vi "SlotValidationA1.vi"(10 "EdgeSlotSides":T3[](array[typedef]) {"Distance (Real-World)" format="%.2f"; "Location (Real-World)"."Y" format="%.2g"; "Location (Real-World)"."X" format="%.2f"; "Noise" format="%.2f"; "Location (Pixel)"."Y" format="%.2g"; "Location (Pixel)"."X" format="%.2f"; "Strength" format="%.2f"; "Distance (Pixel)" format="%.2f"}, 11 "ImageIn":T2) -> (2 "槽点":T1(array[cluster]), 3 "ImageOut":T2)   [LabVIEW 2018]
uses:
  <vilib>/vision/Measure.llb/Edge New.ctl
  <vilib>/vision/Image Controls.llb/IMAQ Image.ctl
  <vilib>/vision/NI_Vision_Development_Module.lvlib
panel:
  out "error in (no error) 2":errorcluster caption="error in (no error)"
  in  "验证取点位置":u32 format="%x"
  in  "error in (no error)":errorcluster
  out "Display Image 3":T2(plugin-control)
  in  "限度-槽内平均亮度-上限":sgl=25.0
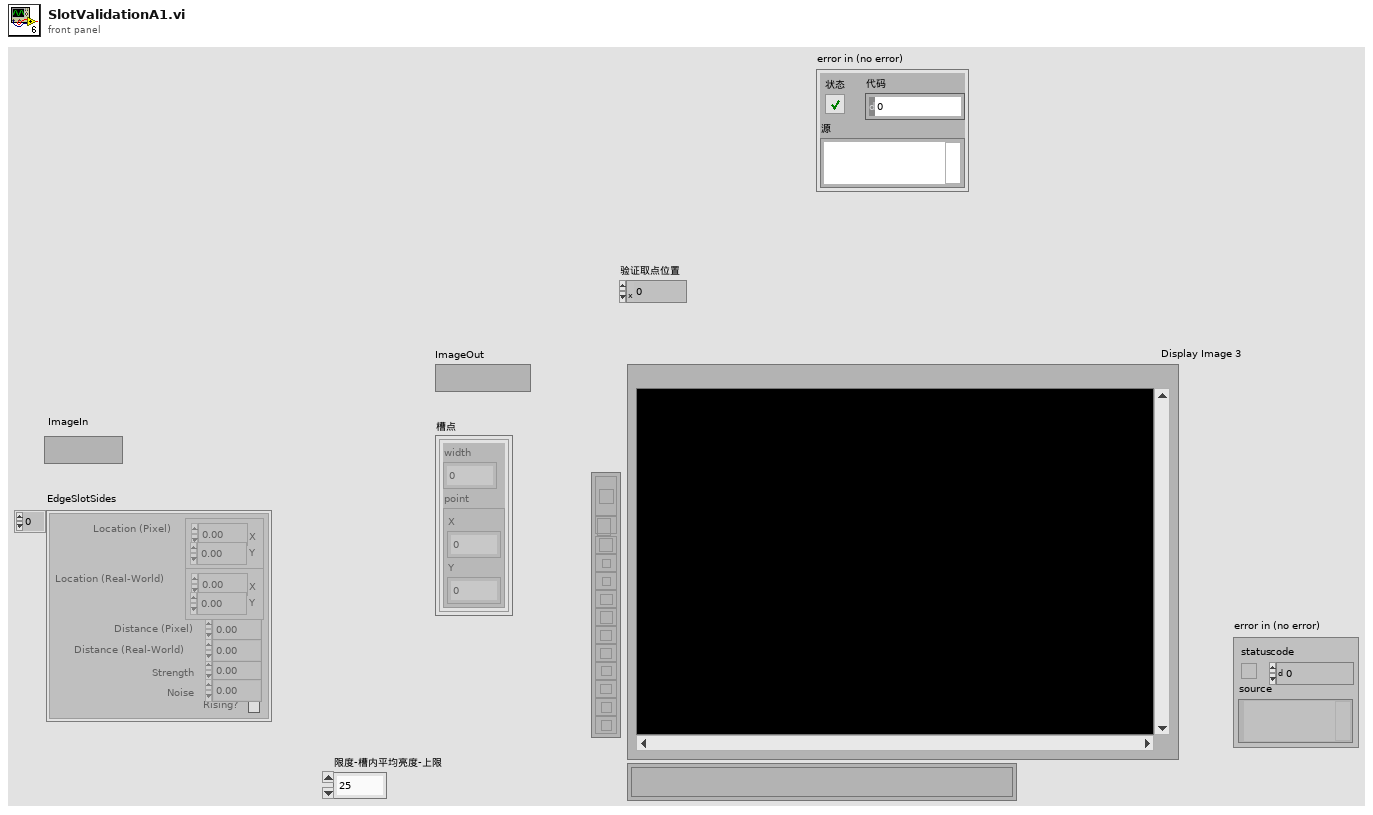
[diagram p1: front panel]
types:
  T1 = cluster{"width":sgl, "point":cluster{"X":sgl, "Y":sgl}}[]
  T2 = typedef "IMAQ Image.ctl" = refnum<image>
  T3 = typedef "Edge New.ctl" = cluster{"Location (Pixel)":cluster{"X":sgl, "Y":sgl}, "Location (Real-World)":cluster{"X":sgl, "Y":sgl}, "Distance (Pixel)":dbl, "Distance (Real-World)":dbl, "Strength":dbl, "Noise":dbl, "Rising?":bool}
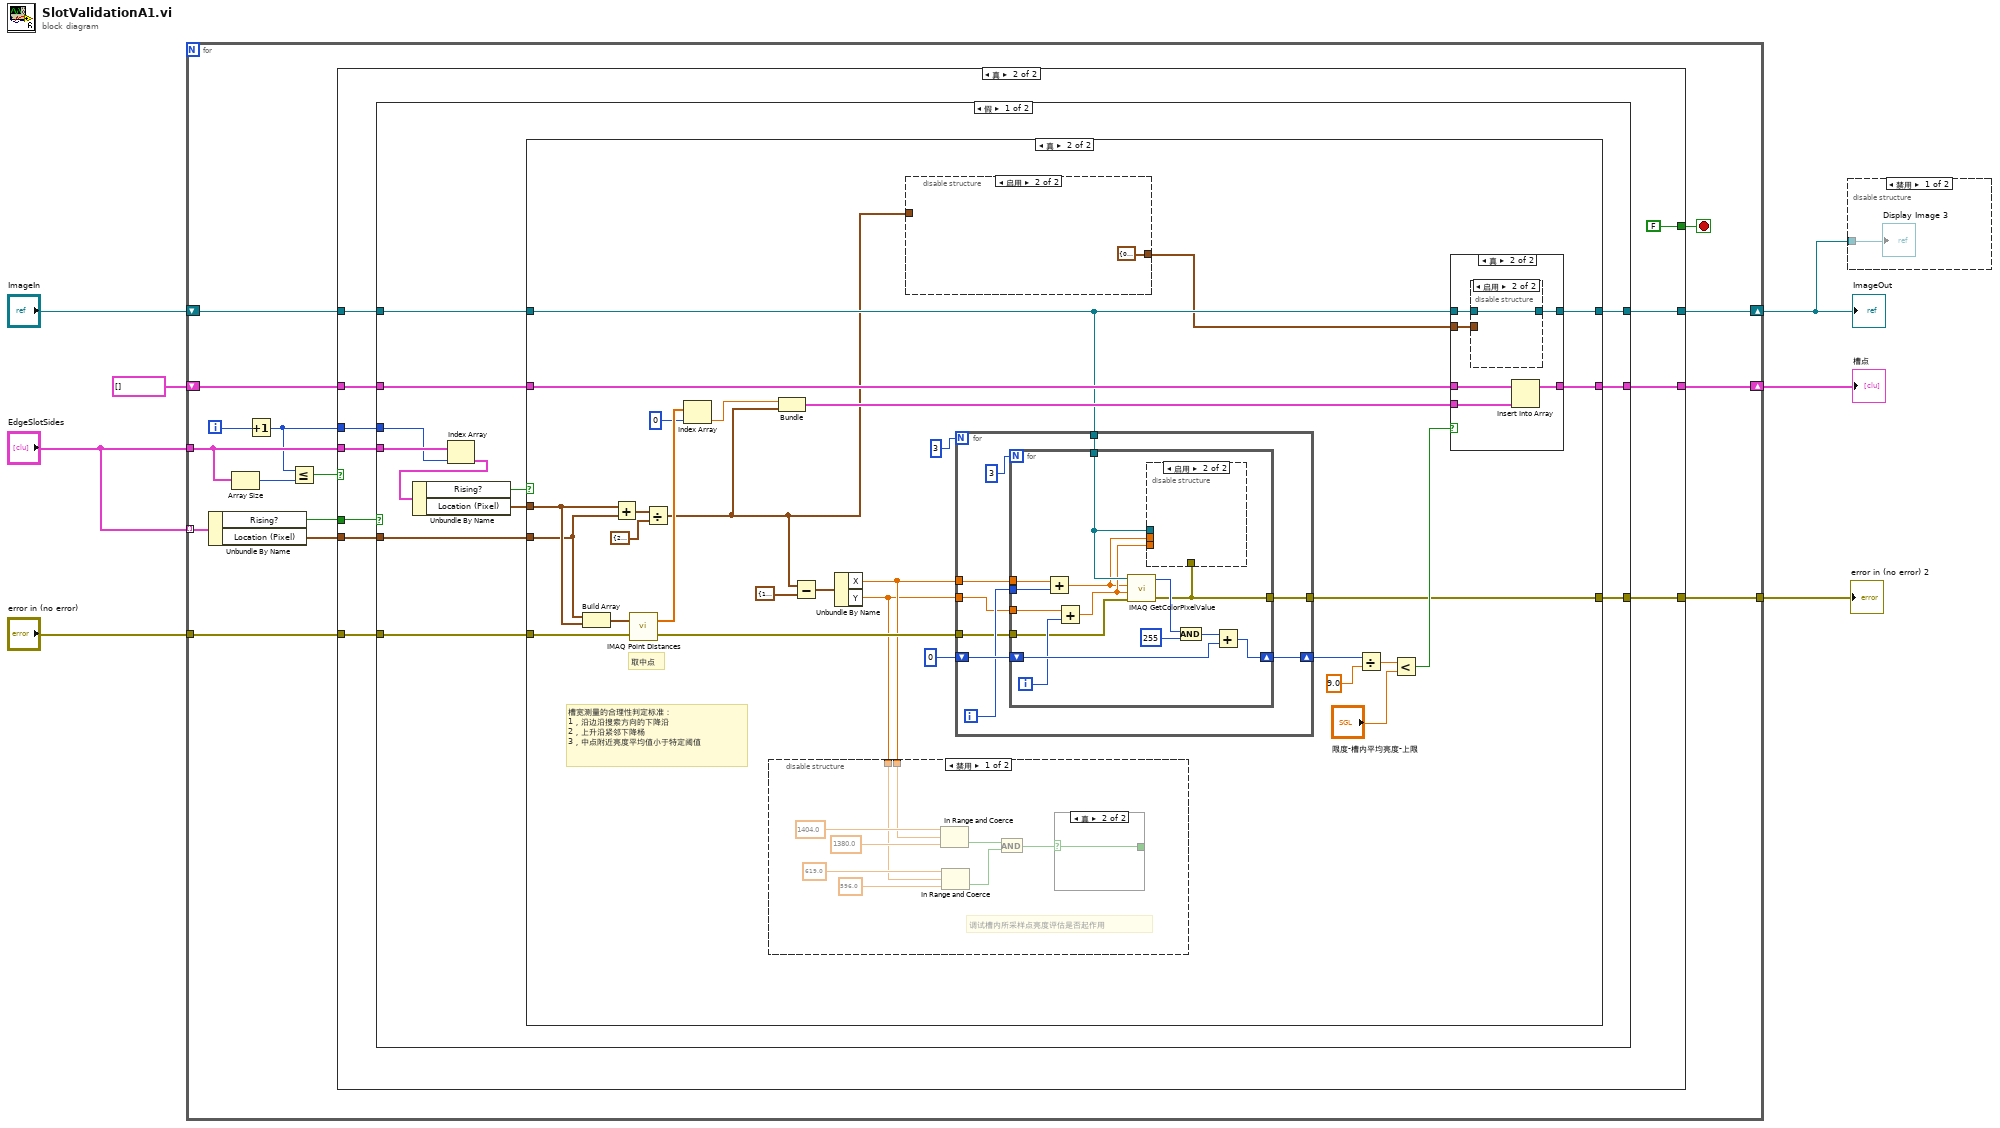
[diagram p0: block diagram]
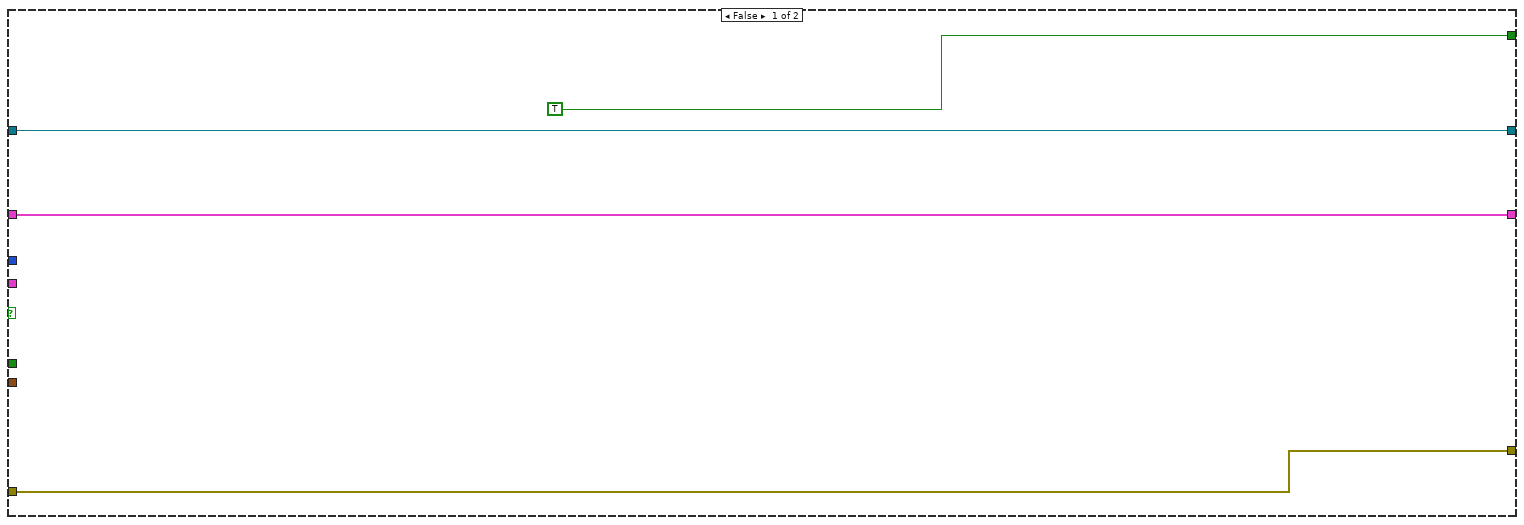
[diagram p3: hidden frame]
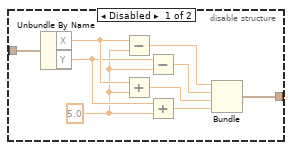
[diagram p7: hidden frame]
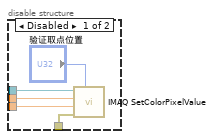
[diagram p8: hidden frame]
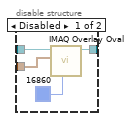
[diagram p10: hidden frame]
diagram:
  n1 = for {
    tunnel: "EdgeSlotSides" -> [w22] mode=indexing
    tunnel: "EdgeSlotSides" -> [w18]
    shift-right: [w13] -> w3
    shift-left: T1 [] ("初始化的数组") -> [w14]
    shift-right: [w11] -> w4
    shift-left: "ImageIn" -> [w12]
    tunnel: "error in (no error)" -> [w9]
    tunnel: [w8] -> w1
    i -> [w19]
    stop <- w15 stop-if-true
    n2 = Unbundle By Name(w22) -> ("Rising?"=w21:bool, "Location (Pixel)"=w20:cluster{"X":sgl, "Y":sgl})
    n3 = Array Size(array=w18) -> (size(s)=w17:i32)
    n4 = Increment(x=w19) -> (x+1=w10:i32)
    n5 = Less Or Equal?(x=w10, y=w17) -> (x <= y?=w16:bool)
    n6 = case shown="真" w16 {
      tunnel: w18 -> [_ w37]
      tunnel: w21 -> [_ w36]
      tunnel: w20 -> [_ w35]
      tunnel: [TRUE FALSE] -> w15
      tunnel: w14 -> [w25 w33]
      tunnel: [w25 w32] -> w13
      tunnel: w12 -> [w24 w31]
      tunnel: [w24 w30] -> w11
      tunnel: w10 -> [_ w29]
      tunnel: w9 -> [w23 w28]
      tunnel: [w23 w27] -> w8
      frame False {
      }
      frame True {
        n7 = case shown="假" w36 {
          tunnel: w37 -> [w49 _]
          tunnel: w35 -> [w45 _]
          tunnel: w33 -> [w44 w146]
          tunnel: [w43 w146] -> w32
          tunnel: w31 -> [w42 w145]
          tunnel: [w41 w145] -> w30
          tunnel: w29 -> [w40 _]
          tunnel: w28 -> [w39 w144]
          tunnel: [w38 w144] -> w27
          frame False {
            n8 = Index Array(array=w49, index=w40) -> (element=w48:T3)
            n9 = Unbundle By Name(w48) -> ("Rising?"=w47:bool, "Location (Pixel)"=w46:cluster{"X":sgl, "Y":sgl})
            n10 = case shown="真" w47 {
              tunnel: w46 -> [_ w69]
              tunnel: w45 -> [_ w68]
              tunnel: w44 -> [w52 w81]
              tunnel: [w52 w80] -> w43
              tunnel: w42 -> [w51 w62]
              tunnel: [w51 w61] -> w41
              tunnel: w39 -> [w50 w60]
              tunnel: [w50 w56] -> w38
              frame False {
              }
              frame True {
                # "槽宽测量的合理性判定标准：\n1，沿边沿搜索方向的下降沿\n2，上升沿紧邻下降杨\n3，中点附近亮度平均值小于特定阈值"
                # "取中点"
                n11 = Build Array(w68, w69) -> (w67:cluster{"X":sgl, "Y":sgl}[])
                n12 = Add(x=w69, y=w68) -> (x+y=w79:cluster{"X":sgl, "Y":sgl})
                n13 = call "IMAQ Point Distances"("Points"=w67, "error in (no error)"=w60) -> ("Distances"=w65:sgl[], "error out"=w59:errorcluster)  [unwired: 3 in]
                n14 = Divide(x=w79, y=cluster{"X":sgl, "Y":sgl} {"X"=2.0, "Y"=2.0} ("Location (Pixel)")) -> (x/y=w55:cluster{"X":sgl, "Y":sgl})
                n15 = Index Array(array=w65, index=0 ("索引")) -> (element=w63:sgl)
                n16 = Bundle(w63, w55) -> (w66:cluster{sgl, cluster{"X":sgl, "Y":sgl}})  [unwired: 1 in]
                n17 = Subtract(x=w55, y=cluster{"X":sgl, "Y":sgl} {"X"=1.0, "Y"=1.0} ("Location (Pixel)")) -> (x-y=w58:cluster{"X":sgl, "Y":sgl})
                n18 = Unbundle By Name(w58) -> ("X"=w54:sgl, "Y"=w53:sgl)
                n19 = disable-structure shown="禁用" {
                  disable-tunnel: w54 -> [w86 _]
                  disable-tunnel: w53 -> [w85 _]
                  frame Disabled {
                    # "调试槽内所采样点亮度评估是否起作用"
                    n20 = In Range and Coerce(upper limit=1404.0 ("上限"), x=w86, lower limit=1380.0 ("下限")) -> (In Range?=w84:bool)  [unwired: 1 out]
                    n21 = In Range and Coerce(upper limit=619.0 ("上限"), x=w85, lower limit=596.0 ("下限")) -> (In Range?=w83:bool)  [unwired: 1 out]
                    n22 = And(x=w84, y=w83) -> (x .and. y?=w82:bool)
                    n23 = case shown="真" w82 {
                      selector: w82 -> [w91 w92]
                      tunnel: [w91 w92] -> _
                      frame False {
                      }
                      frame True {
                      }
                    }
                  }
                  frame Enabled {
                  }
                }
                n24 = disable-structure shown="启用" {
                  disable-tunnel: [w94 cluster{sgl, sgl, sgl, sgl} {0.0, 0.0, 0.0, 0.0}] -> w57
                  disable-tunnel: w55 -> [w93 _]
                  frame Disabled {
                    w96 = sgl 5.0 ("y")
                    n25 = Unbundle By Name(w93) -> ("X"=w99:sgl, "Y"=w97:sgl)
                    n26 = Subtract(x=w99, y=w96) -> (x-y=w101:sgl)
                    n27 = Add(x=w99, y=w96) -> (x+y=w98:sgl)
                    n28 = Subtract(x=w97, y=w96) -> (x-y=w100:sgl)
                    n29 = Add(x=w97, y=w96) -> (x+y=w95:sgl)
                    n30 = Bundle(w101, w100, w98, w95) -> (w94:cluster{sgl, sgl, sgl, sgl})  [unwired: 1 in]
                  }
                  frame Enabled {
                  }
                }
                n31 = for {
                  N: 3 -> [_]
                  shift-right: [w108] -> w74
                  shift-left: u32 0 ("Pixel Value (U32)") -> [w109]
                  tunnel: w62 -> [w110]
                  tunnel: w54 -> [w107]
                  tunnel: w53 -> [w105]
                  tunnel: w59 -> [w104]
                  tunnel: [w103] -> w56
                  i -> [w106]
                  n32 = for {
                    N: 3 -> [_]
                    shift-right: [w121] -> w108
                    shift-left: w109 -> [w122]
                    tunnel: w110 -> [w115]
                    tunnel: w107 -> [w120]
                    tunnel: w106 -> [w119]
                    tunnel: w105 -> [w118]
                    tunnel: w104 -> [w116]
                    tunnel: [w112] -> w103
                    i -> [w117]
                    n33 = Add(x=w120, y=w119) -> (x+y=w113:sgl)
                    n34 = Add(x=w118, y=w117) -> (x+y=w114:sgl)
                    n35 = call "IMAQ GetColorPixelValue"("error in (no error)"=w116, "Y Coordinate"=w114, "X Coordinate"=w113, "Image"=w115) -> ("error out"=w112:errorcluster, "Pixel Value (U32)"=w125:u32)  [unwired: 1 out]
                    n36 = disable-structure shown="启用" {
                      disable-tunnel: w115 -> [w130 _]
                      disable-tunnel: w112 -> [w129 _]
                      disable-tunnel: w114 -> [w128 _]
                      disable-tunnel: w113 -> [w127 _]
                      frame Disabled {
                        n37 = call "IMAQ SetColorPixelValue"("Pixel Value (U32)"="验证取点位置", "error in (no error)"=w129, "Y Coordinate"=w128, "X Coordinate"=w127, "Image"=w130) -> ()  [unwired: 5 in, 2 out]
                      }
                      frame Enabled {
                      }
                    }
                    n38 = And(x=w125, y=u32 255) -> (x .and. y?=w123:u32)
                    n39 = Add(x=w123, y=w122) -> (x+y=w121:u32)
                  }
                }
                n40 = Divide(x=w74, y=9.0) -> (x/y=w70:dbl)
                n41 = Less?(x=w70, y="限度-槽内平均亮度-上限") -> (x < y?=w76:bool)
                n42 = case shown="真" w76 {
                  tunnel: w81 -> [w132 w138]
                  tunnel: [w132 w137] -> w80
                  tunnel: w66 -> [_ w136]
                  tunnel: w62 -> [w131 w135]
                  tunnel: [w131 w134] -> w61
                  tunnel: w57 -> [_ w133]
                  frame False {
                  }
                  frame True {
                    n43 = disable-structure shown="启用" {
                      disable-tunnel: w135 -> [w142 w143]
                      disable-tunnel: [w141 w143] -> w134
                      disable-tunnel: w133 -> [w140 _]
                      frame Disabled {
                        n44 = call "IMAQ Overlay Oval"("Color"=u32 16860, "Bounding Rectangle"=w140, "Image"=w142) -> ("Image Out"=w141:T2)  [unwired: 7 in, 1 out]
                      }
                      frame Enabled {
                      }
                    }
                    n45 = Insert Into Array(array=w138, new element=w136) -> (w137:T1)  [unwired: 1 in]
                  }
                }
              }
            }
          }
          frame True {
          }
        }
      }
    }
  }
  "ImageOut" <- w4
  "槽点" <- w3
  "error in (no error) 2" <- w1
  n46 = disable-structure shown="禁用" {
    disable-tunnel: w4 -> [w147 _]
    frame Disabled {
      "Display Image 3" <- w147
    }
    frame Enabled {
    }
  }
